vi "record one experiment.vi"(7 "Exp. file path":path, 8 "error in":errorcluster, 11 "Sample index":i32) -> (0 "error in 2":errorcluster)   [LabVIEW 2017]
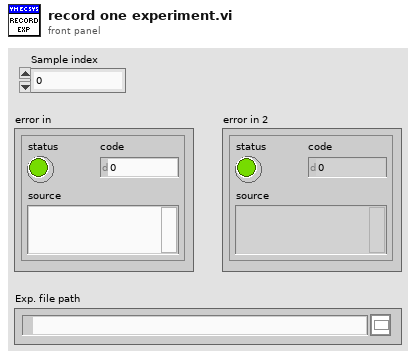
[diagram p1: front panel]
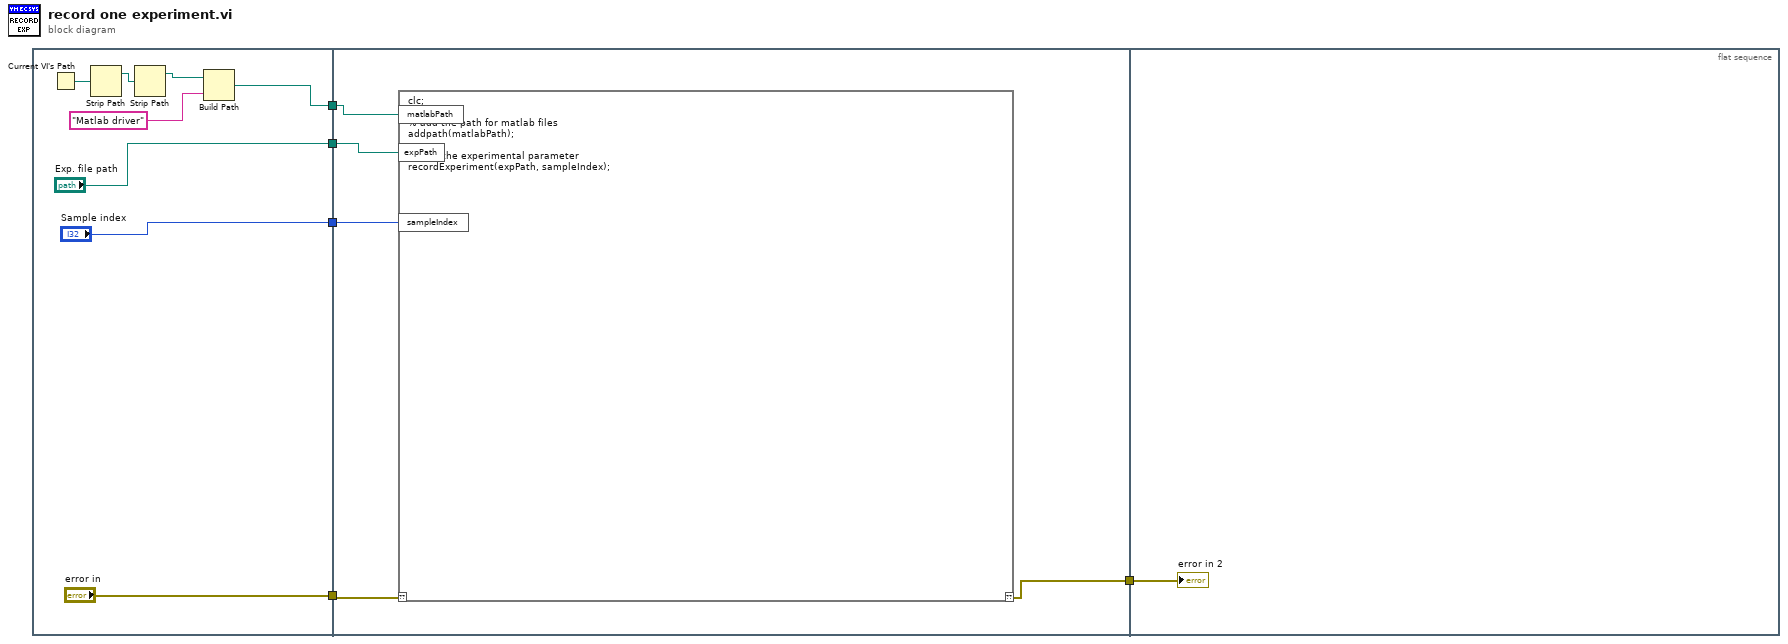
[diagram p0: block diagram]
diagram:
  n1 = flat-sequence {
    tunnel: [w9] -> w5
    tunnel: ["error in"] -> w4
    tunnel: ["Exp. file path"] -> w3
    tunnel: ["Sample index"] -> w1
    tunnel: w5 -> [w18]
    tunnel: w4 -> [w16]
    tunnel: w3 -> [w17]
    tunnel: [w15] -> w2
    tunnel: w1 -> [w14]
    tunnel: w2 -> [w19]
    frame #0 {
      n2 = Current VI's Path() -> (path=w13:path)
      n3 = Strip Path(path=w13) -> (stripped path=w11:path)  [unwired: 1 out]
      n4 = Strip Path(path=w11) -> (stripped path=w10:path)  [unwired: 1 out]
      n5 = Build Path(base path=w10, name or relative path="Matlab driver") -> (appended path=w9:path)
    }
    frame #1 {
      n6 = script code="clc;\n\n% add the path for matlab files\naddpath(matlabPath);\n\n%read the experimental parameter\nrecordExperiment(expPath, sampleIndex);"("??"=w16, "matlabPath"=w18, "expPath"=w17, "sampleIndex"=w14) -> ("??"=w15:errorcluster)
    }
    frame #2 {
      "error in 2" <- w19
    }
  }
